vi "Global FTT Display.vi"(8 "error in (no error)":errorcluster, 10 "W/R":bool, 11 "Display":T1) -> (0 "error out":errorcluster, 3 "Display OUT":T1)   [LabVIEW 2014]
uses:
  Type'def/FTT Display Type.ctl
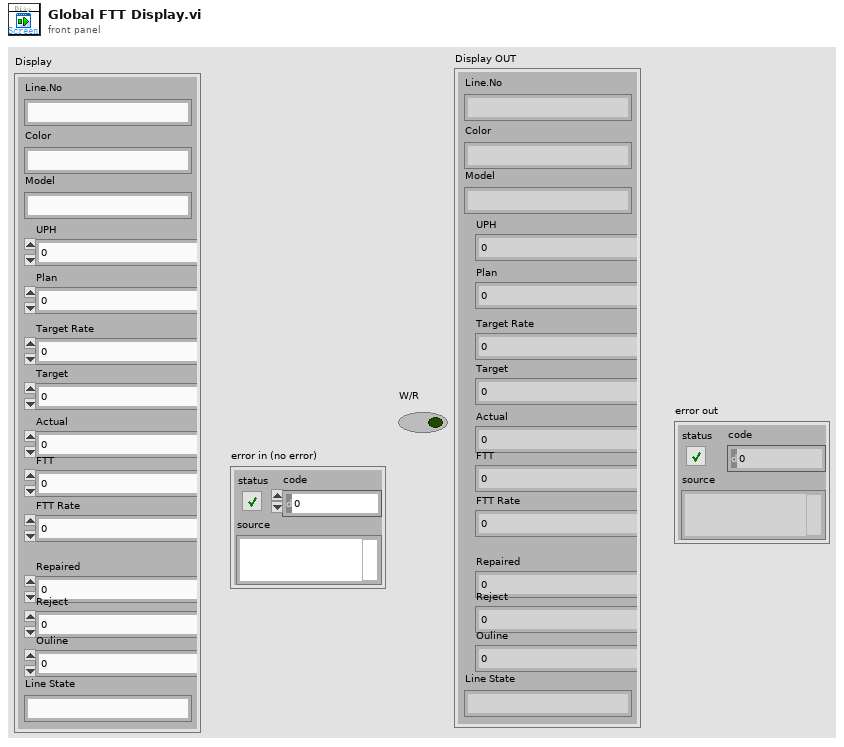
[diagram p1: front panel]
types:
  T1 = typedef "FTT Display Type.ctl" = cluster{"Line.No":string, "Model":string, "Color":string, "UPH":dbl, "Plan":dbl, "Target Rate":dbl, "Target ":dbl, "Actual":dbl, "FTT":dbl, "FTT Rate":dbl, "Repaired":dbl, "Reject":dbl, "Ouline":dbl, "Line State":string}
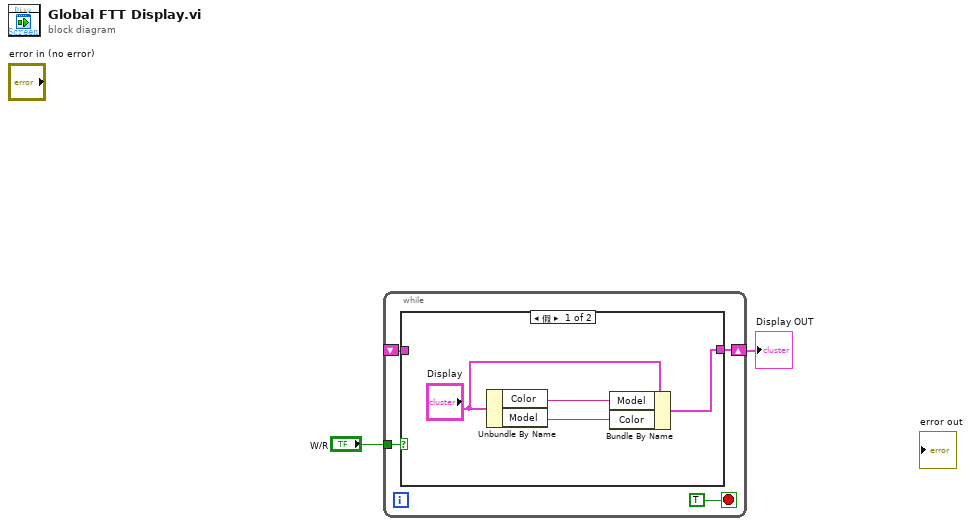
[diagram p0: block diagram]
diagram:
  n1 = while {
    tunnel: "W/R" -> [w5]
    shift-right: [w4] -> w1
    shift-left: _ -> [w3]
    stop <- TRUE stop-if-true
    n2 = case shown="假" w5 {
      tunnel: [w9 w11] -> w4
      tunnel: w3 -> [_ w11]
      frame False {
        n3 = Unbundle By Name("Display") -> ("Color"=w8:string, "Model"=w7:string)
        n4 = Bundle By Name(cluster="Display", "Model"=w8, "Color"=w7) -> (w9:T1)
      }
      frame True {
      }
    }
  }
  "Display OUT" <- w1
